vi "000EH_电导率_温度偏移修正值写入.vi"(8 "error in (no error)":errorcluster caption="错误输入（无错误）", 10 "数值":sgl, 11 "MB_Serial session in":refnum<class "MB_Master_Serial.lvclass">) -> (0 "error out":errorcluster caption="错误输出", 3 "MB_Serial session out":refnum<class "MB_Master_Serial.lvclass">)   [LabVIEW 2016, in "斯坦道多参数.lvlib"]
uses:
  <vilib>/Plasmionique/MB Master/MB_Master_Serial/MB_Master_Serial.lvclass
  C:/Program Files (x86)/National Instruments/LabVIEW 2016/vi.lib/Plasmionique/MB Master/MB_Master/MB_Master.lvclass
  <vilib>/Plasmionique/MB Master/MB Master.lvlib
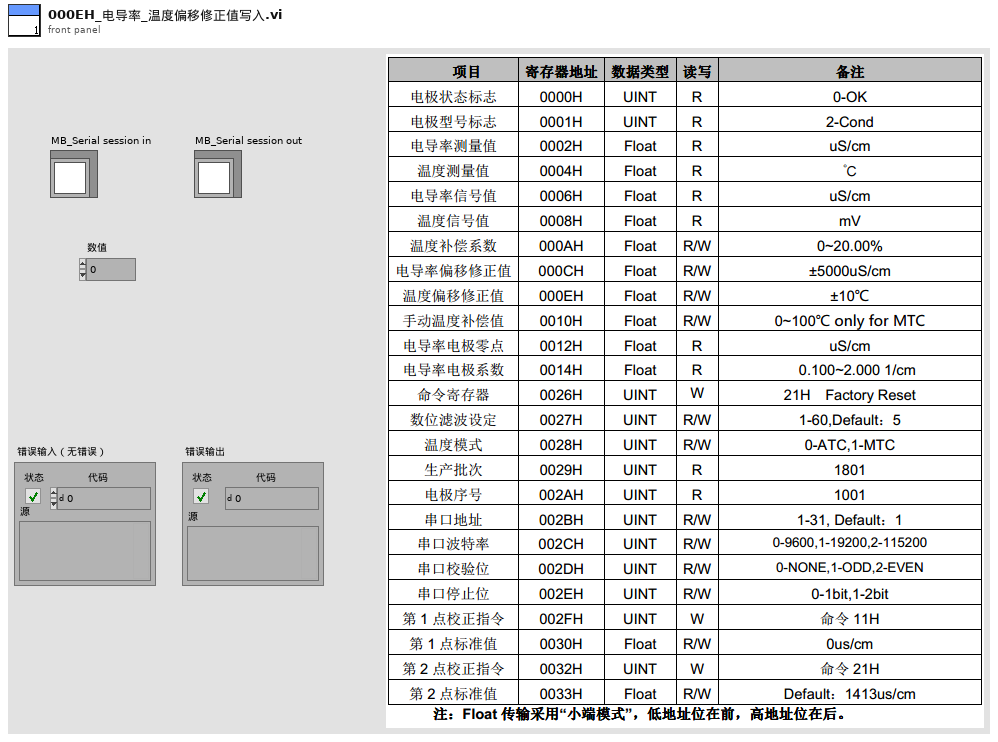
[diagram p1: front panel]
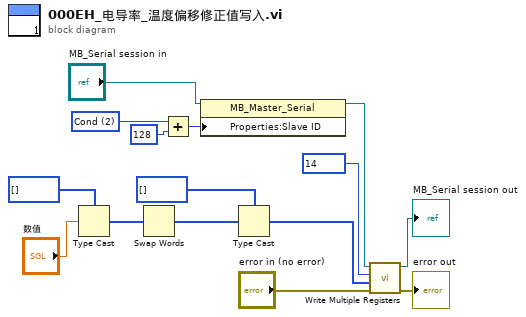
[diagram p0: block diagram]
diagram:
  w8 = u16 2 items=["NULL", "pH", "Cond", "DO", "Turb"] ("数值")
  n1 = Type Cast(type=u32[] [] ("数组 2"), x="数值") -> (*(type *) &x=w9:u32[])
  n2 = Swap Words(1:w9) -> (0:w2:u32[])
  n3 = Add(x=w8, y=u16 128) -> (x+y=w7:u16)
  n4 = property class="MB_Master_Serial"(reference="MB_Serial session in", "Properties:Slave ID"=w7) -> (reference out=w4:refnum<class "MB_Master_Serial.lvclass">)  [unwired: 1 in, 1 out]
  n5 = Type Cast(type=u16[] [] ("数组 2"), x=w2) -> (*(type *) &x=w1:u16[])
  n6 = call <vilib>:"Write Multiple Registers.vi"("error in (no error)"="error in (no error)", "values"=w1, "starting address"=u16 14, "MB session in"=w4) -> ("error out"=→"error out":errorcluster, "MB session out"=→"MB_Serial session out":refnum<class "MB_Master_Serial.lvclass">)  [unwired: 6 in]
